vi "SimulationAndDataOverlay.vi"() -> ()   [LabVIEW 2014]
uses:
  <vilib>/Utility/file.llb/Read From Spreadsheet File (DBL).vi
panel:
  out "all rows":dbl[][](array[numeric]) format="%0.3f"
  in  "Path":path=path "U:/phys 434/week8/Shaken5minData"
  out "Waveform Chart":dbl[][](graph)=[[2.3666654058215677], [3.0]]
  out "Waveform Graph":dbl[][](graph)
  out "best fit":dynamicdata(graph)=[{"t0"=timestamp(0 s since 1904-01-01), "dt"=1.0, "Y"=array[302 elements], "attributes"=variant("NI_ChannelName"=variant(string "Best fit"))}]
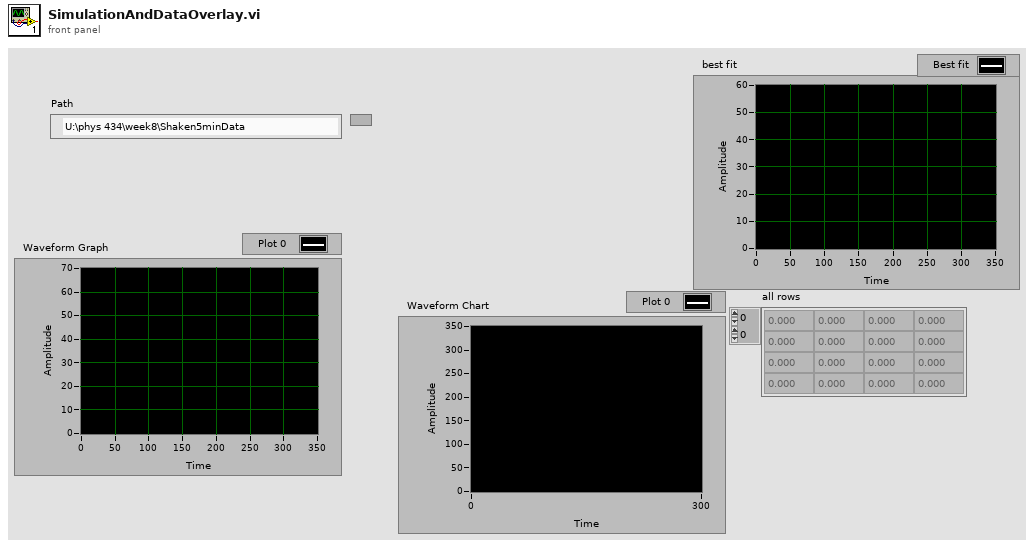
[diagram p1: front panel]
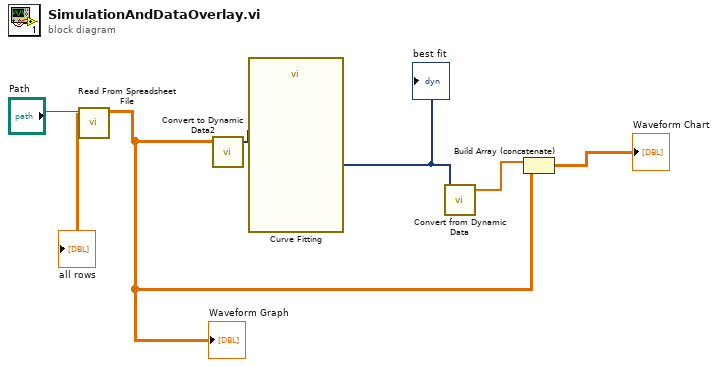
[diagram p0: block diagram]
diagram:
  n1 = call-poly <vilib>:"Read From Spreadsheet File.vi"("file path (dialog if empty)"="Path") -> ("all rows"=w1:dbl[][])  [unwired: 6 in, 4 out]
  "Waveform Graph" <- w1
  "all rows" <- w1
  n2 = call "Convert to Dynamic Data2"("2D Array"=w1) -> ("Dynamic Data Type"=w3:dynamicdata)  [unwired: 3 in]
  n3 = call "Curve Fitting"("Signals"=w3) -> ("best fit"=w6:dynamicdata)  [unwired: 6 in, 4 out]
  "best fit" <- w6
  n4 = call "Convert from Dynamic Data"("Dynamic Data Type"=w6) -> ("Array"=w5:dbl[])  [unwired: 3 in]
  n5 = Build Array (concatenate)(w5, w1) -> (→"Waveform Chart":dbl[][])
